vi "Prepare Inputs.vi"(7 "SMO":refnum<class "SMO.lvclass">, 8 "error in (no error)":errorcluster, 10 "Inputs":variant, 11 "API":T1) -> (0 "error out":errorcluster, 3 "API dup":T1)   [LabVIEW 2013, in "SMOFacade.lvlib" / "SMOFacade.lvclass"]
uses:
  SMOFacade.lvclass
  Registry/SMO_API--Cluster.ctl
  Terminal/Terminal.lvclass
  SMO/SMO.lvclass
  Registry/Registry-SMO.lvclass
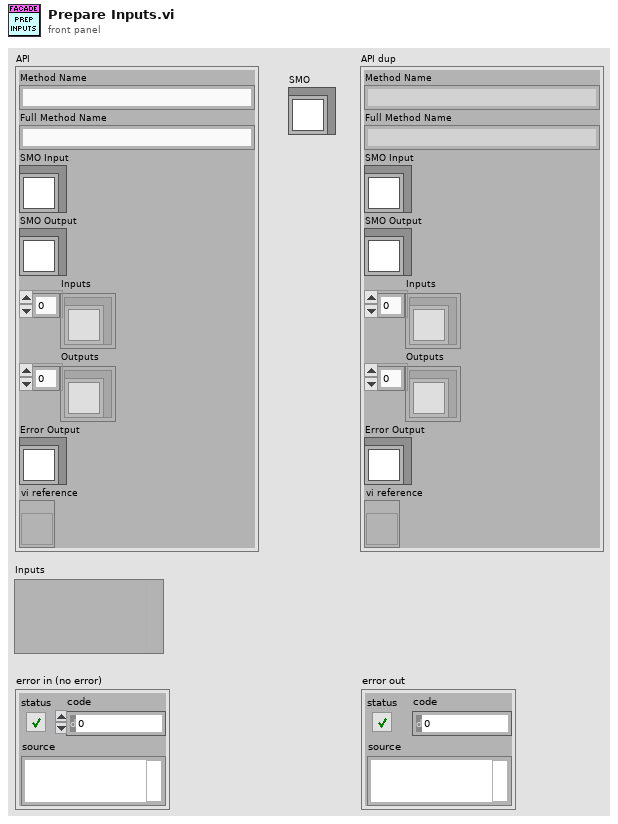
[diagram p1: front panel]
types:
  T1 = typedef "Registry-SMO.lvclass/SMO_API--Cluster.ctl" = cluster{"Method Name":string, "Full Method Name":string, "SMO Input":refnum<class "Terminal.lvclass">, "SMO Output":refnum<class "Terminal.lvclass">, "Inputs":refnum<class "Terminal.lvclass">[], "Outputs":refnum<class "Terminal.lvclass">[], "Error Output":refnum<class "Terminal.lvclass">, "vi reference":refnum<vi>}
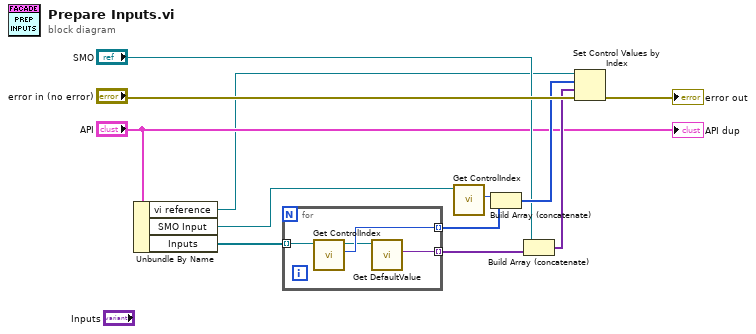
[diagram p0: block diagram]
diagram:
  n1 = Unbundle By Name("API") -> ("vi reference"=w1:refnum<vi>, "SMO Input"=w10:refnum<class "Terminal.lvclass">, "Inputs"=w4:refnum<class "Terminal.lvclass">[])
  n2 = for {
    tunnel: w4 -> [w16] mode=indexing
    tunnel: [w15] -> w9 mode=indexing
    tunnel: [w14] -> w8 mode=indexing
    n3 = call "Get ControlIndex.vi"("Terminal in"=w16) -> ("ControlIndex"=w15:i32, "Terminal out"=w13:refnum<class "Terminal.lvclass">)  [unwired: 8 in, 1 out]
    n4 = call "Get DefaultValue.vi"("Terminal in"=w13) -> ("Default Value"=w14:variant)  [unwired: 7 in, 3 out]
  }
  n5 = call "Get ControlIndex.vi"("Terminal in"=w10) -> ("ControlIndex"=w11:i32)  [unwired: 8 in, 2 out]
  n6 = Build Array (concatenate)(w11, w9) -> (w6:i32[])
  n7 = Build Array (concatenate)("SMO", w8) -> (w7:variant[])
  n8 = Set Control Values by Index(0:w1, 1:w6, 2:w7, 3:"error in (no error)") -> (11:→"error out":errorcluster)
  "API dup" <- "API"
